vi "FPGA Personality(9040).vi"   [LabVIEW 2020]
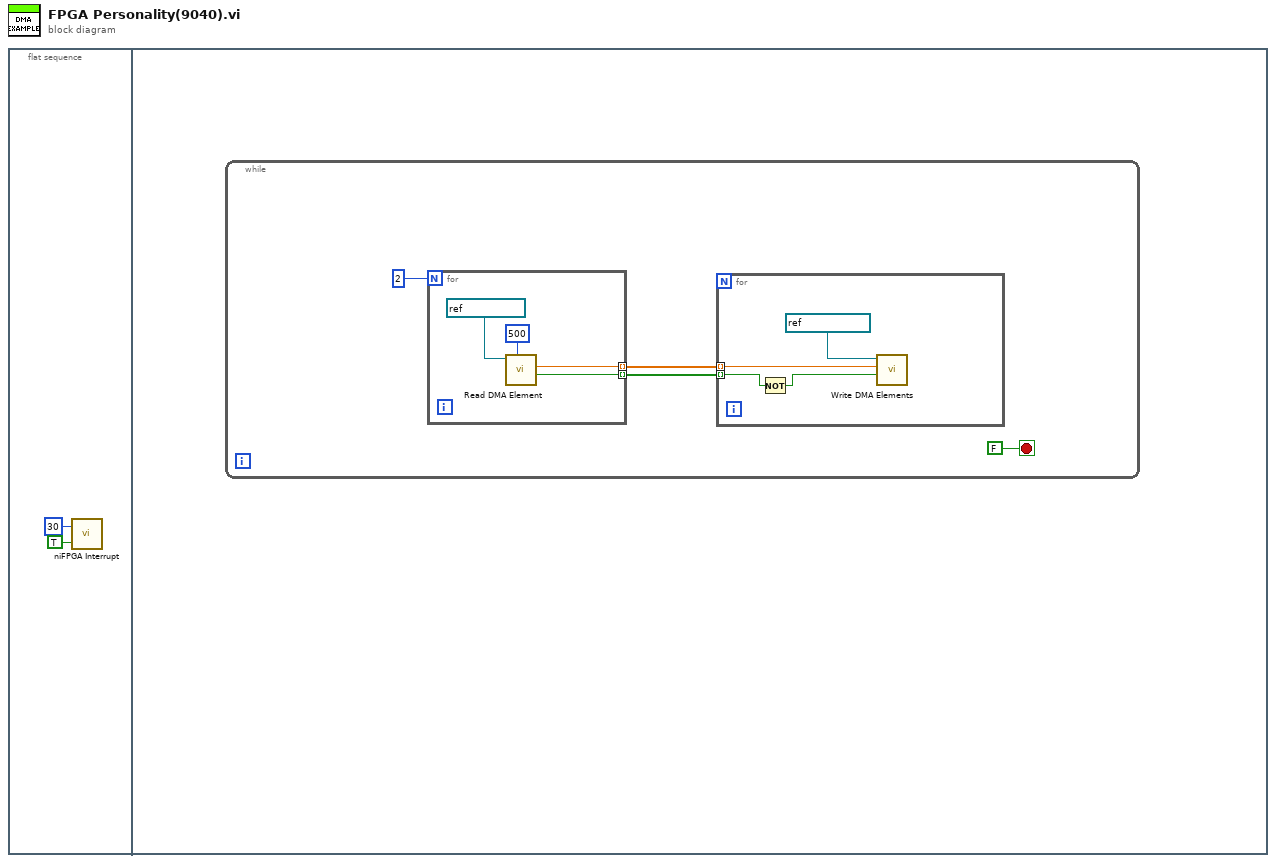
[diagram p0: block diagram]
diagram:
  n1 = flat-sequence {
    frame #0 {
      n2 = call <vilib>:"niFPGA Interrupt.vi"("Wait Until Cleared (F)"=TRUE, "IRQ Number (0)"=u8 30) -> ()  [unwired: 1 in]
    }
    frame #1 {
      n3 = while {
        stop <- FALSE stop-if-true
        n4 = for {
          N: 2 -> [_]
          tunnel: [w12] -> w4 mode=indexing
          tunnel: [w11] -> w3 mode=indexing
          n5 = call "Read DMA Element.vi"("Timeout"=500, "DMA Refnum in"=refnum<k21> "Incoming" ("FIFO In")) -> ("isTimeout ?"=w11:bool, "DMA Element"=w12:sgl)  [unwired: 7 in, 1 out]
        }
        n6 = for {
          tunnel: w4 -> [w8] mode=indexing
          tunnel: w3 -> [w7] mode=indexing
          n7 = Not(x=w7) -> (.not. x?=w9:bool)
          n8 = call "Write DMA Elements.vi"("isValid ?"=w9, "DMA Element"=w8, "FIFO Refnum in"=refnum<k21> "Outgoing2" ("FIFO In")) -> ()  [unwired: 8 in, 1 out]
        }
      }
    }
  }
